vi "marshalling.vi"(8 "error in (no error)":errorcluster, 10 "Variant":variant, 11 "Serializer":refnum<class "Serializer.PlainText.INI.lvclass">) -> (0 "error out":errorcluster, 2 "String":string, 3 "Serializer out":refnum<class "Serializer.PlainText.INI.lvclass">)   [LabVIEW 2013, in "Serializer.PlainText.INI.lvclass"]
uses:
  Serializer.PlainText.INI.lvclass
  <vilib>/LabVIEW Open Source Project/Data Manipulation/TypeDescriptor/TypeDescriptor_GetName.vi
  <vilib>/LabVIEW Open Source Project/Data Manipulation/TypeDescriptor/TypeDescriptor_GetPString.vi
  <vilib>/Utility/GetType.llb/Get Type Code from I16 Array And Pos.vi
  <vilib>/Utility/GetType.llb/TD_Get Array Information.vi
  <vilib>/LabVIEW Open Source Project/Data Manipulation/TypeDescriptor/TypeDescriptor_SetName.vi
  <vilib>/LabVIEW Open Source Project/Data Manipulation/Variant/OpenVariant.lvlib
  <vilib>/Utility/VariantDataType/VariantType.lvlib
  Serializer.PlainText/Serializer.PlainText.lvclass
  <vilib>/LabVIEW Open Source Project/Data Manipulation/TypeDescriptor/OpenDescriptor.lvlib
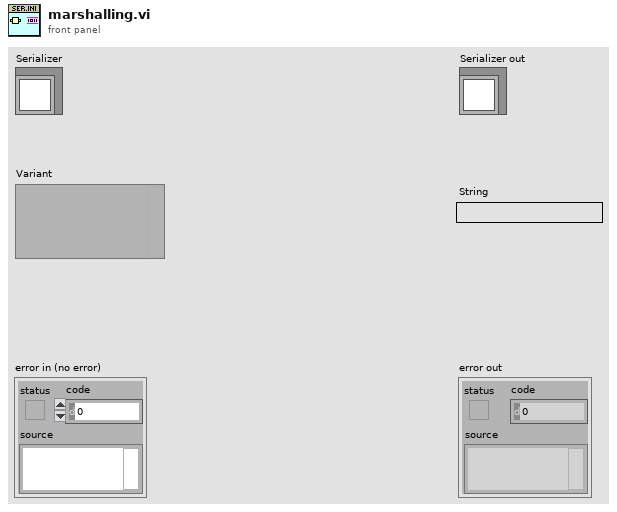
[diagram p1: front panel]
types:
  T1 = typedef "VariantType.lvlib/Type.ctl" = enum8{"Invalid Type", "Void", "I8", "I16", "I32", "I64", "U8", "U16", "U32", "U64", "Single Float", "Double Float", "Extended Float", "Single Complex", "Double Complex", "Extended Complex", "Enum U8", "Enum U16", "Enum U32", "Enum U64", "Single Float With Unit", "Double Float With Unit", "Extended Float With Unit", "Single Complex with Unit", "Double Complex with Unit", "Extended Complex with Unit", "Boolean", "String", "Path", "Picture", "Tag", "Array", "Cluster", "Variant", "LV Variant", "Waveform", "Timestamp", "Digital Waveform", "Digital Data", "ExpressData", "Refnum", "External Data", "VI", "Poly VI", "LabVIEW Class Instance", "Fixed Point"}
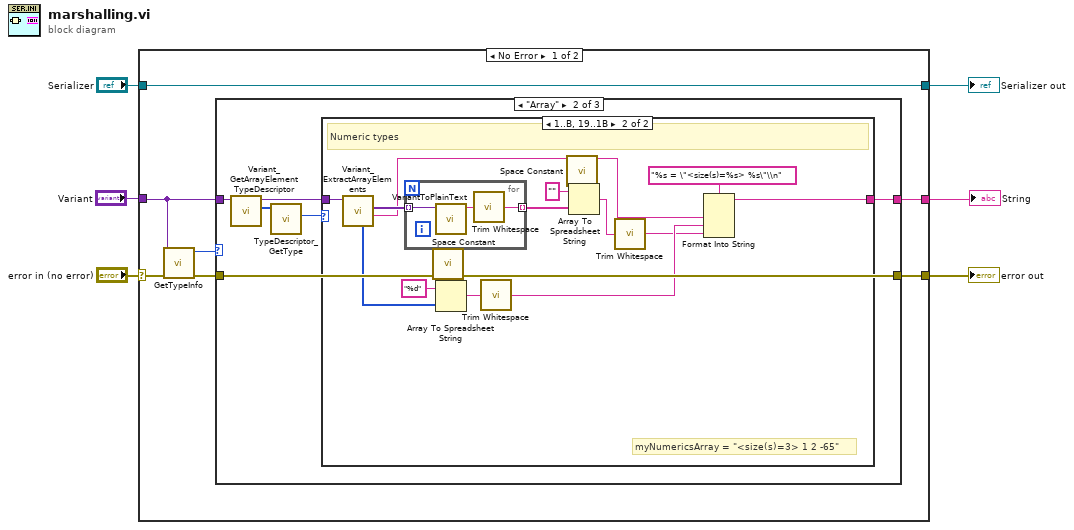
[diagram p0: block diagram]
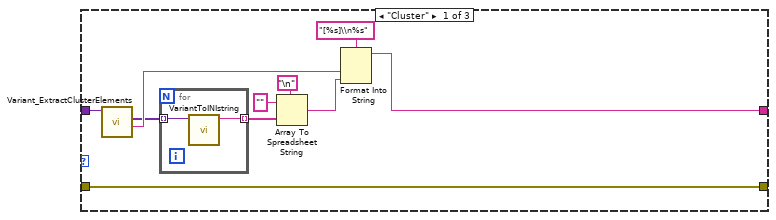
[diagram p2: hidden frame]
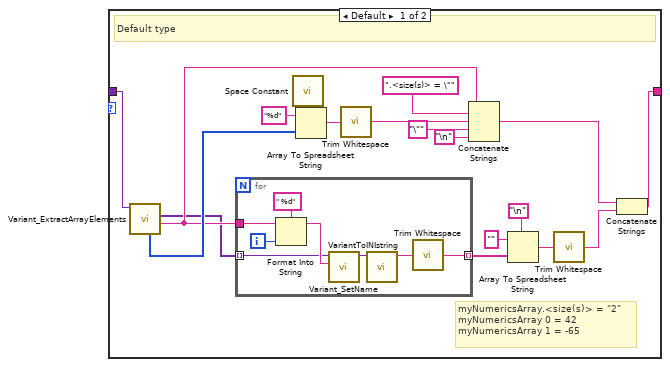
[diagram p3: hidden frame]
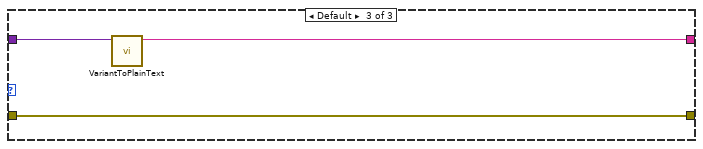
[diagram p4: hidden frame]
diagram:
  n1 = case shown="No Error" "error in (no error)" {
    selector: "error in (no error)" -> [w11 w80]
    tunnel: [w8 w80] -> w5
    tunnel: [w13 w79] -> w3
    tunnel: "Serializer" -> [w13 w79]
    tunnel: "Variant" -> [w7 _]
    tunnel: [w12 _] -> w1
    frame No Error {
      n2 = call <vilib>:"GetTypeInfo.vi"("error in (no error)"=w11, "Variant"=w7) -> ("error out"=w9:errorcluster, "Type Enum"=w10:T1)  [unwired: 5 in, 3 out]
      n3 = case shown="\"Array\"" w10 {
        tunnel: [w16 w28 w76] -> w12
        tunnel: w7 -> [w15 w27 w77]
        tunnel: w9 -> [w14 w26 w78]
        tunnel: [w14 w26 w78] -> w8
        frame "Cluster" {
          n4 = call <vilib>:"Variant_ExtractClusterElements.vi"("Cluster"=w15) -> ("name"=w21:string, "Elements"=w17:variant[])  [unwired: 8 in, 1 out]
          n5 = for {
            tunnel: [w25] -> w20 mode=indexing
            tunnel: w17 -> [w24] mode=indexing
            n6 = call "VariantToINIstring.vi"("Variant-formatted Value"=w24) -> ("String-formatted Value"=w25:string)  [unwired: 10 in]
          }
          n7 = Array To Spreadsheet String(delimiter (Tab)="\n", array=w20, 3:"" ("format string")) -> (spreadsheet string=w23:string)
          n8 = Format Into String(format string="[%s]\\n%s", w21, w23) -> (resulting string=w16:string)  [unwired: 2 in, 1 out]
        }
        frame "Array" {
          n9 = call <vilib>:"Variant_GetArrayElementTypeDescriptor.vi"("Array"=w27) -> ("Element Descriptor"=w31:i16[], "Array dup"=w30:variant)  [unwired: 8 in, 1 out]
          n10 = call <vilib>:"TypeDescriptor_GetType.vi"("type descriptor"=w31) -> ("Type"=w29:u8)  [unwired: 9 in, 1 out]
          n11 = case shown="1..B, 19..1B" w29 {
            tunnel: [w49 w60] -> w28
            tunnel: w30 -> [w32 w64]
            frame Default {
              # "myNumericsArray.<size(s)> = \"2\"\nmyNumericsArray 0 = 42\nmyNumericsArray 1 = -65"
              # "Default type"
              n12 = call <vilib>:"Variant_ExtractArrayElements.vi"("Array"=w32) -> ("name"=w39:string, "Elements"=w38:variant[], "Dimensions"=w45:u32[])  [unwired: 7 in, 1 out]
              n13 = for {
                tunnel: w39 -> [w54]
                tunnel: w38 -> [w50] mode=indexing
                tunnel: [w51] -> w35 mode=indexing
                i -> [w56]
                n14 = Format Into String(format string=" %d" ("Format String"), initial string=w54, w56) -> (resulting string=w53:string)  [unwired: 1 in, 1 out]
                n15 = call <vilib>:"Variant_SetName.vi"("Name"=w53, "Variant"=w50) -> ("Named Variant"=w55:variant)  [unwired: 9 in]
                n16 = call "VariantToINIstring.vi"("Variant-formatted Value"=w55) -> ("String-formatted Value"=w52:string)  [unwired: 10 in]
                n17 = call <vilib>:"Trim Whitespace.vi"("string"=w52) -> ("trimmed string"=w51:string)  [unwired: 1 in]
              }
              n18 = call <vilib>:"Space Constant.vi"() -> ("String"=w48:string)
              n19 = Array To Spreadsheet String(delimiter (Tab)=w48, array=w45, 3:"%d" ("format string")) -> (spreadsheet string=w46:string)
              n20 = call <vilib>:"Trim Whitespace.vi"("string"=w46) -> ("trimmed string"=w41:string)  [unwired: 1 in]
              n21 = Concatenate Strings(w39, ".<size(s)> = \"" ("Substring"), w41, "\"" ("string"), "\n") -> (w40:string)
              n22 = Array To Spreadsheet String(delimiter (Tab)="\n", array=w35, 3:"" ("format string")) -> (spreadsheet string=w34:string)
              n23 = call <vilib>:"Trim Whitespace.vi"("string"=w34) -> ("trimmed string"=w33:string)  [unwired: 1 in]
              n24 = Concatenate Strings(w40, w33) -> (w49:string)
            }
            frame 1..11, 25..27 {
              # "myNumericsArray = \"<size(s)=3> 1 2 -65\""
              # "Numeric types"
              n25 = call <vilib>:"Variant_ExtractArrayElements.vi"("Array"=w64) -> ("name"=w58:string, "Elements"=w68:variant[], "Dimensions"=w69:u32[])  [unwired: 7 in, 1 out]
              n26 = for {
                tunnel: w68 -> [w74] mode=indexing
                tunnel: [w75] -> w66 mode=indexing
                n27 = call "VariantToPlainText.vi"("Variant-formatted Value"=w74) -> ("String-formatted Value"=w73:string)  [unwired: 10 in]
                n28 = call <vilib>:"Trim Whitespace.vi"("string"=w73) -> ("trimmed string"=w75:string)  [unwired: 1 in]
              }
              n29 = call <vilib>:"Space Constant.vi"() -> ("String"=w72:string)
              n30 = Array To Spreadsheet String(delimiter (Tab)=w72, array=w69, 3:"%d" ("format string")) -> (spreadsheet string=w70:string)
              n31 = call <vilib>:"Trim Whitespace.vi"("string"=w70) -> ("trimmed string"=w62:string)  [unwired: 1 in]
              n32 = call <vilib>:"Space Constant.vi"() -> ("String"=w59:string)
              n33 = Array To Spreadsheet String(delimiter (Tab)=w59, array=w66, 3:"" ("format string")) -> (spreadsheet string=w65:string)
              n34 = call <vilib>:"Trim Whitespace.vi"("string"=w65) -> ("trimmed string"=w61:string)  [unwired: 1 in]
              n35 = Format Into String(format string="%s = \"<size(s)=%s> %s\"\\n", w58, w62, w61) -> (resulting string=w60:string)  [unwired: 2 in, 1 out]
            }
          }
        }
        frame Default {
          n36 = call "VariantToPlainText.vi"("Variant-formatted Value"=w77) -> ("String-formatted Value"=w76:string)  [unwired: 10 in]
        }
      }
    }
    frame Error {
    }
  }
  "error out" <- w5
  "Serializer out" <- w3
  "String" <- w1
